vi "Encoder.vi"() -> ()   [LabVIEW 2021]
panel:
  in  "CounterSize":enum32{"8Bits", "16Bits", "32Bits"}(radio)
  in  "EncodeType":enum32{"X1", "X2", "X4"}(radio)
  in  "Stop":bool
  out "TotalDistance":dbl format="%#.2f"
  out "Gauge":dbl(knob) scale=0.0..360.0
  in  "WheelDiameter":dbl=770.0
  # "cm"
  # "meters"
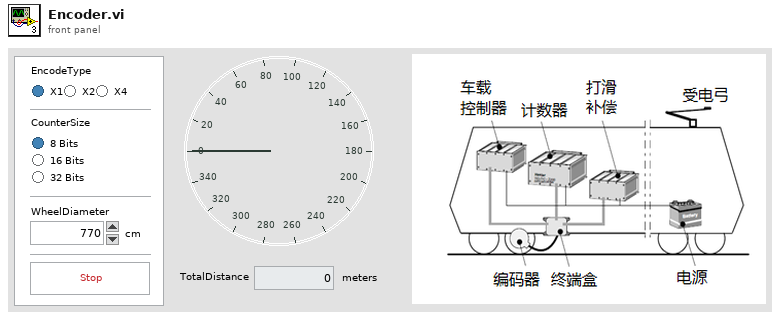
[diagram p1: front panel]
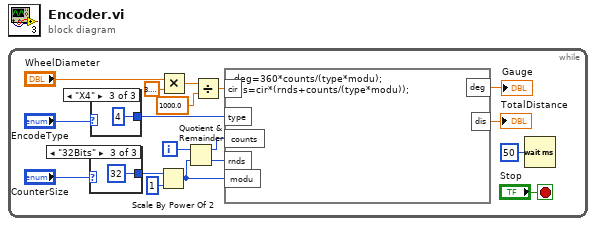
[diagram p0: block diagram]
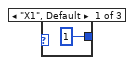
[diagram p2: hidden frame]
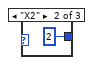
[diagram p3: hidden frame]
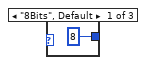
[diagram p4: hidden frame]
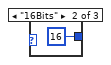
[diagram p5: hidden frame]
diagram:
  n1 = while {
    i -> [w12]
    stop <- "Stop" stop-if-true
    n2 = case shown="\"32Bits\"" "CounterSize" {
      tunnel: [u32 8 ("n") u32 16 ("n") u32 32 ("n")] -> w17
      frame "8Bits", Default {
      }
      frame "16Bits" {
      }
      frame "32Bits" {
      }
    }
    n3 = case shown="\"X4\"" "EncodeType" {
      tunnel: [u32 1 ("n") u32 2 ("n") u32 4 ("n")] -> w16
      frame "X1", Default {
      }
      frame "X2" {
      }
      frame "X4" {
      }
    }
    n4 = Scale By Power Of 2(n=w17, x=u32 1) -> (x*2^n=w6:u32)
    n5 = Multiply(x="WheelDiameter", y=3.141592653589793) -> (x*y=w7:dbl)
    n6 = Quotient & Remainder(x=w12, y=w6) -> (x-y*floor(x/y)=w11:u32, floor(x/y)=w10:u32)
    n7 = Divide(x=w7, y=1000.0) -> (x/y=w5:dbl)
    n8 = formula code="deg=360*counts/(type*modu);\ndis=cir*(rnds+counts/(type*modu));"("type"=w16, "counts"=w11, "rnds"=w10, "cir"=w5, "modu"=w6) -> ("deg"=→"Gauge":dbl, "dis"=→"TotalDistance":dbl)
    n9 = Wait (ms)(milliseconds to wait=u32 50) -> ()  [unwired: 1 out]
  }
